vi "Get LabVIEW Files.vi"(8 "error in (no error)":errorcluster, 10 "LabVIEW File Type":T1, 11 "Session in":refnum<class "Session.lvclass">) -> (0 "error out":errorcluster, 2 "LabVIEW Files":refnum<class "LabVIEW File.lvclass">[](array[class]), 3 "Session out":refnum<class "Session.lvclass">)   [LabVIEW 2020, in "Save for Previous Version.lvlib" / "Session.lvclass"]
uses:
  Session.lvclass
  Session.lvclass/Session.ctl
  LabVIEW File/LabVIEW File.lvclass
  File/File.lvclass/File.lvclass
  <vilib>/Utility/lvfile.llb/FT_FileTypes.ctl
  <vilib>/Utility/lvfile.llb/NI_FileType.lvlib
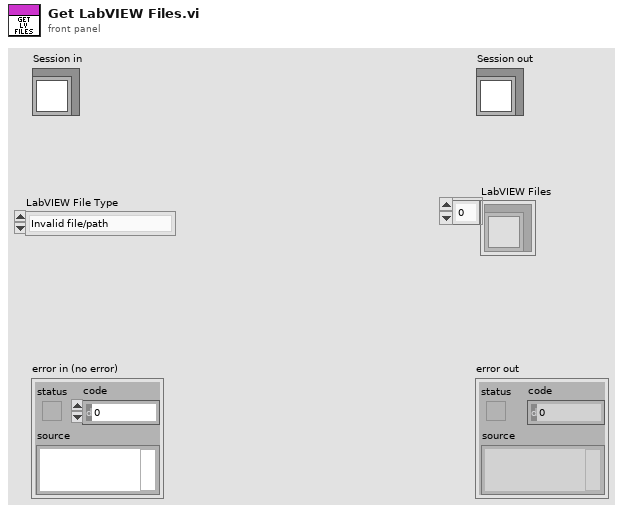
[diagram p1: front panel]
types:
  T1 = typedef "NI_FileType.lvlib/FT_FileTypes.ctl" = enum32{"Invalid file/path", "Unknown type", "Instrument", "Control", "Polymorphic VI", "Project", "Library", "LVClass", "XControl", "XNode", "CIN", "Run-time menu", "Palette menu", "LLB", "Shortcut", "Directory", "Class Private Data Control", "Statechart", "MathScript .m file", "Ladder Diagram", "LVLibp"}
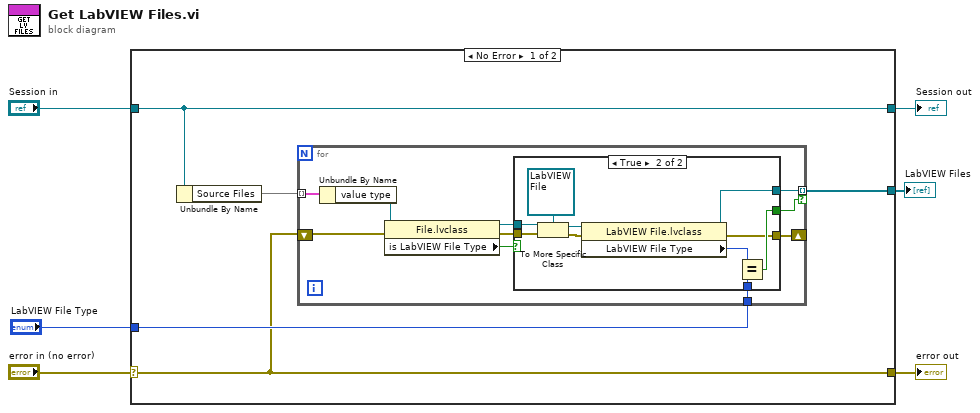
[diagram p0: block diagram]
diagram:
  n1 = case shown="No Error" "error in (no error)" {
    selector: "error in (no error)" -> [w7 w34]
    tunnel: [w7 w34] -> w5
    tunnel: [w11 w33] -> w3
    tunnel: "Session in" -> [w11 w33]
    tunnel: "LabVIEW File Type" -> [w9 _]
    tunnel: [w8 _] -> w1
    frame No Error {
      n2 = Unbundle By Name(w11) -> ("Source Files"=w10:map{path, refnum<class "File.lvclass">})
      n3 = for {
        tunnel: w10 -> [w13] mode=indexing
        tunnel: w9 -> [w20]
        tunnel: [w14] -> w8 mode=indexing if=w19
        shift-right: [w15] -> _
        shift-left: w7 -> [w17]
        n4 = Unbundle By Name(w13) -> ("value type"=w12:refnum<class "File.lvclass">)
        n5 = property class="File.lvclass"(reference=w12, error in=w17) -> (reference out=w21:refnum<class "File.lvclass">, error out=w16:errorcluster, "is LabVIEW File Type"=w18:bool)
        n6 = case shown="True" w18 {
          tunnel: w21 -> [_ w32]
          tunnel: w20 -> [_ w28]
          tunnel: [_ w26] -> w14
          tunnel: [_ w25] -> w19
          tunnel: w16 -> [w22 w24]
          tunnel: [w22 w23] -> w15
          frame False {
          }
          frame True {
            n7 = To More Specific Class(target class=refnum<class "LabVIEW File.lvclass"> refnum ("Save for Previous Version.lvlib:LabVIEW File.lvclass"), reference=w32, error in=w24) -> (specific class reference=w29:refnum<class "LabVIEW File.lvclass">, error out=w30:errorcluster)
            n8 = property class="LabVIEW File.lvclass"(reference=w29, error in=w30) -> (reference out=w26:refnum<class "LabVIEW File.lvclass">, error out=w23:errorcluster, "LabVIEW File Type"=w27:T1)
            n9 = Equal?(x=w27, y=w28) -> (x = y?=w25:bool)
          }
        }
      }
    }
    frame Error {
    }
  }
  "error out" <- w5
  "Session out" <- w3
  "LabVIEW Files" <- w1
